vi "Actor Core.vi"(8 "error in":errorcluster, 11 "root_actor in":refnum<class "root_actor.lvclass">) -> (0 "error out":errorcluster, 3 "Actor out":refnum<class "Actor.lvclass">)   [LabVIEW 2025, in "root_actor.lvlib" / "root_actor.lvclass"]
doc: "(<B>Filename</B>: Actor Framework.lvlib:Actor.lvclass:Actor Core.vi)\n\nReceives messages to the actor, reacts to them, and initiates any error handling that may shut the actor down.\n\nDescendant classes may override this VI to append parallel tasks for the actor to complete while it handles messages. Overrides use the Call Parent Class Method node."
uses:
  root_actor.lvclass
  <vilib>/ActorFramework/Actor/Actor.lvclass
  <vilib>/ActorFramework/Message Enqueuer/Message Enqueuer.lvclass
  root_actor.lvclass/root_actor.ctl
  Udate Nested Attributes Messages/update_attrs Msg/update_attrs Msg.lvclass/update_attrs Msg.ctl
  <vilib>/ActorFramework/Message Enqueuer/Message Enqueuer.lvclass/Message Enqueuer.ctl
  <vilib>/ActorFramework/Message Enqueuer/Enqueue.vi
  Udate Nested Attributes Messages/update_attrs Msg/update_attrs Msg.lvclass
  <vilib>/ActorFramework/Message Priority Queue/Priority Enqueue.vi
  <vilib>/regexp/Match Regular Expression.xnode
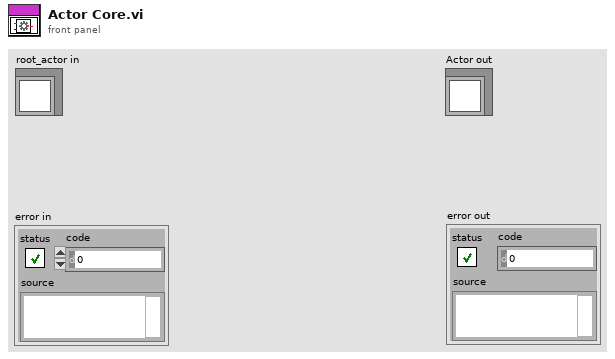
[diagram p1: front panel]
types:
  T1 = map{string, refnum<class "Message Enqueuer.lvclass">}
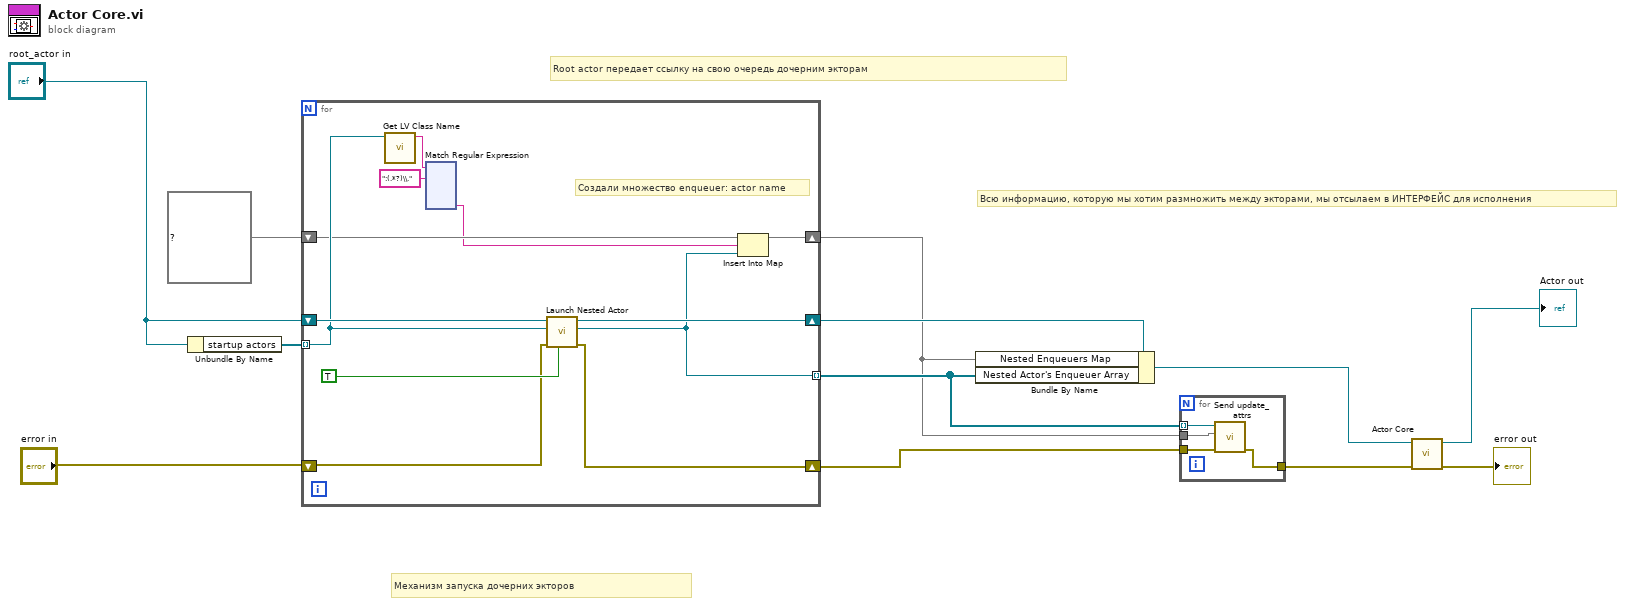
[diagram p0: block diagram]
diagram:
  # "Всю информацию, которую мы хотим размножить между экторами, мы отсылаем в ИНТЕРФЕЙС для исполнения"
  # "Root actor передает ссылку на свою очередь дочерним экторам"
  # "Механизм запуска дочерних экторов"
  n1 = Unbundle By Name("root_actor in") -> ("startup actors"=w9:refnum<class "Actor.lvclass">[])
  n2 = for {
    tunnel: w9 -> [w17] mode=indexing
    shift-right: [w23] -> w8
    shift-left: "root_actor in" -> [w24]
    tunnel: [w15] -> w2 mode=indexing
    shift-right: [w20] -> w4
    shift-left: "error in" -> [w21]
    shift-right: [w13] -> w1
    shift-left: T1 {} ("map") -> [w16]
    # "Создали множество enqueuer: actor name"
    n3 = call <vilib>:"Get LV Class Name.vi"("object"=w17) -> ("class name"=w19:string)  [unwired: 9 in, 1 out]
    n4 = xnode "Match Regular Expression"("input string"=w19, "regular expression"=":(.*?)\\.") -> ("submatch 1"=w14:string)  [unwired: 4 in, 5 out]
    n5 = call <vilib>:"Launch Nested Actor.vi"("Open Actor Core front panel? (F)"=TRUE, "error in (no error)"=w21, "Nested Actor"=w17, "Caller Actor in"=w24) -> ("error out"=w20:errorcluster, "Nested Actor's Enqueuer"=w15:refnum<class "Message Enqueuer.lvclass">, "Caller Actor out"=w23:refnum<class "root_actor.lvclass">)  [unwired: 5 in]
    n6 = Insert Into Map(map in=w16, key=w14, value=w15) -> (map out=w13:T1)  [unwired: 2 out]
  }
  n7 = Bundle By Name(cluster=w8, "Nested Enqueuers Map"=w1, "Nested Actor's Enqueuer Array"=w2) -> (w5:refnum<class "root_actor.lvclass">)
  n8 = for {
    tunnel: w4 -> [w147]
    tunnel: [w146] -> w3
    tunnel: w2 -> [w145] mode=indexing
    tunnel: w1 -> [w144]
    n9 = call "Send update_attrs.vi"("error in (no error)"=w147, "Nested Enqueuers Map"=w144, "Message Enqueuer"=w145) -> ("error out"=w146:errorcluster)  [unwired: 7 in, 1 out]
  }
  n10 = call-parent "Actor Core.vi"("error in"=w3, "Actor in"=w5) -> ("error out"=→"error out":errorcluster, "Actor out"=→"Actor out":refnum<class "Actor.lvclass">)  [unwired: 8 in]
